vi "NI_FPGA_PPG.ProcDestructor.vi"(0 "i ref in":refnum<vi>, 3 "ms timeout (10000)":i32=10000, 5 "error in (no error)":errorcluster) -> (14 "i ref out":refnum<vi>, 17 "timed out":bool, 19 "error out":errorcluster)   [LabVIEW 2014, in "NI_FPGA_PPG.lvlib"]
doc: "This method contains some code that needs to be called while executing the destructor."
uses:
  NI_FPGA_PPG.lvlib
  CSlibraries-extern/DimLVEvent/LVDimInterface/LVDimInterface.lvlib
  instr.lib/NI-FPGA-PPG/host/instrumentDriver/NI-FPGA-PPG_Driver.lvlib
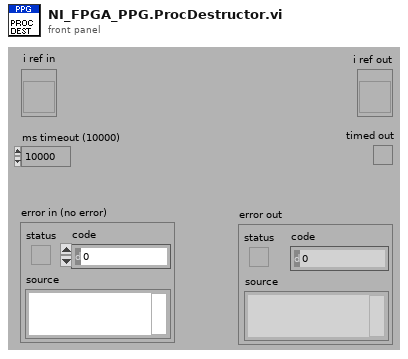
[diagram p1: front panel]
types:
  T1 = typedef "NI_FPGA_PPG.lvlib/NI_FPGA_PPG.i attribute.ctl" = cluster{"dim_service_id":cluster{"dim_actual_device_status":i32, "dim_event_data":i32, "dim_cmd_data":i32, "dim_cmd_data _description":i32, "dim_channel_description":i32}, "VISA":refnum<visa-resource-name>, "actual_device_status":i32, "event_data_id":i32, "pdc_enabled":bool, "pdc_timestamp":u32, "cmd_data_string":string, "cmd_data_size":i32, "cmd_data_description_string":string, "cmd_data_description_size":i32, "channel_description_string":string, "channel_description_size":i32}
  T2 = cluster{"dim_actual_device_status":i32, "dim_event_data":i32, "dim_cmd_data":i32, "dim_cmd_data _description":i32, "dim_channel_description":i32}
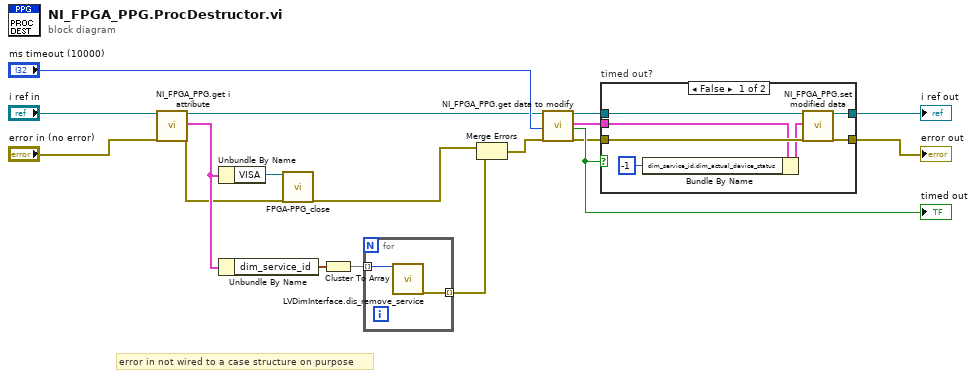
[diagram p0: block diagram]
diagram:
  # "error in not wired to a case structure on purpose"
  n1 = call "NI_FPGA_PPG.get i attribute.vi"("i ref in"="i ref in", "error in (no error)"="error in (no error)") -> ("i ref out"=w10:refnum<vi>, "i attribute"=w11:T1, "error out"=w4:errorcluster)  [unwired: 15 in]
  n2 = Unbundle By Name(w11) -> ("VISA"=w12:refnum<visa-resource-name>)
  n3 = Unbundle By Name(w11) -> ("dim_service_id"=w6:T2)
  n4 = call "FPGA-PPG_close.vi"("resource_in"=w12, "error in (no error)"=w4) -> ("error out"=w1:errorcluster)  [unwired: 17 in]
  n5 = Cluster To Array(cluster=w6) -> (array=w5:i32[])
  n6 = for {
    tunnel: [w20] -> w3 mode=indexing
    tunnel: w5 -> [w19] mode=indexing
    n7 = call "LVDimInterface.dis_remove_service.vi"("my_serviceID"=w19) -> ("error out"=w20:errorcluster)  [unwired: 18 in]
  }
  n8 = Merge Errors(w1, w3) -> (w2:errorcluster)
  n9 = call "NI_FPGA_PPG.get data to modify.vi"("i ref in"=w10, "ms timeout (10000)"="ms timeout (10000)", "error in (no error)"=w2) -> ("i ref out"=w8:refnum<vi>, "i attribute"=w7:T1, "timed out"=w13:bool, "error out"=w9:errorcluster)  [unwired: 13 in]
  "timed out" <- w13
  n10 = case "timed out?" shown="False" w13 {
    tunnel: w9 -> [w26 w28]
    tunnel: w8 -> [w27 w29]
    tunnel: w7 -> [w23 _]
    tunnel: [w25 w29] -> w16
    tunnel: [w24 w28] -> w15
    frame False {
      n11 = Bundle By Name(cluster=w23, "dim_service_id.dim_actual_device_status"=-1 ("_deviceState")) -> (w22:T1)
      n12 = call "NI_FPGA_PPG.set modified data.vi"("i ref in"=w27, "i attribute"=w22, "error in (no error)"=w26) -> ("i ref out"=w25:refnum<vi>, "error out"=w24:errorcluster)  [unwired: 15 in]
    }
    frame True {
    }
  }
  "error out" <- w15
  "i ref out" <- w16
